vi "Close.vi"(8 "error in (no error)":errorcluster, 11 "Interaction in":refnum<class "Interaction.lvclass">) -> (0 "error out":errorcluster)   [LabVIEW 2013, in "Interaction.lvclass"]
doc: "Copyright 2018, Wiebe Walstra, wiebe@carya.nl."
uses:
  Interaction.lvclass
  Interaction.lvclass/Interaction.ctl
  Interaction Splitter.lvclass
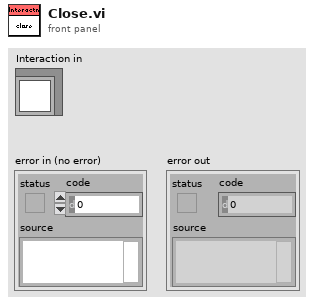
[diagram p1: front panel]
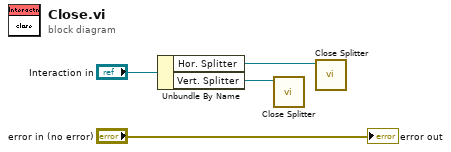
[diagram p0: block diagram]
diagram:
  n1 = Unbundle By Name("Interaction in") -> ("Hor. Splitter"=w2:refnum<class "Interaction Splitter.lvclass">, "Vert. Splitter"=w1:refnum<class "Interaction Splitter.lvclass">)
  n2 = call-dynamic "Close Splitter.vi"("Interaction Splitter in"=w1) -> ()  [unwired: 10 in, 1 out]
  n3 = call-dynamic "Close Splitter.vi"("Interaction Splitter in"=w2) -> ()  [unwired: 10 in, 1 out]
  "error out" <- "error in (no error)"
